vi "Spread.vi"(10 "Input":dbl, 11 "Threshold":dbl=1600.0) -> (3 "spread greater then Vth":bool)   [LabVIEW 2012]
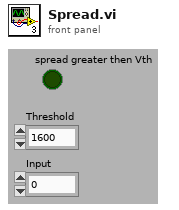
[diagram p1: front panel]
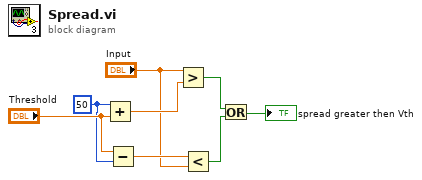
[diagram p0: block diagram]
diagram:
  w6 = 50
  n1 = Add(x=w6, y="Threshold") -> (x+y=w8:dbl)
  n2 = Subtract(x="Threshold", y=w6) -> (x-y=w5:dbl)
  n3 = Greater?(x="Input", y=w8) -> (0:w3:bool)
  n4 = Less?(x=w5, y="Input") -> (x < y?=w2:bool)
  n5 = Or(x=w3, y=w2) -> (x .or. y?=→"spread greater then Vth":bool)
